vi "Click Cycle.vi"(6 "Prior Property Selection":T1(array[cluster]), 7 "Action":T2, 8 "Shift":bool, 9 "Coords":cluster{"Horizontal":i32, "Vertical":i32}, 10 "All Tree Refs":refnum<vi>[](array[refnum]), 11 "Tree Control Ref":refnum<vi>) -> (0 "Error Out":errorcluster, 2 "Clicked disabled item?":bool)   [LabVIEW 2023]
doc: "Toggle symbol (R/W) for clicked items in tree."
uses:
  controls/action enum.ctl
panel:
  out "Tag Selected":string[](array[string])
  in  "error in":errorcluster
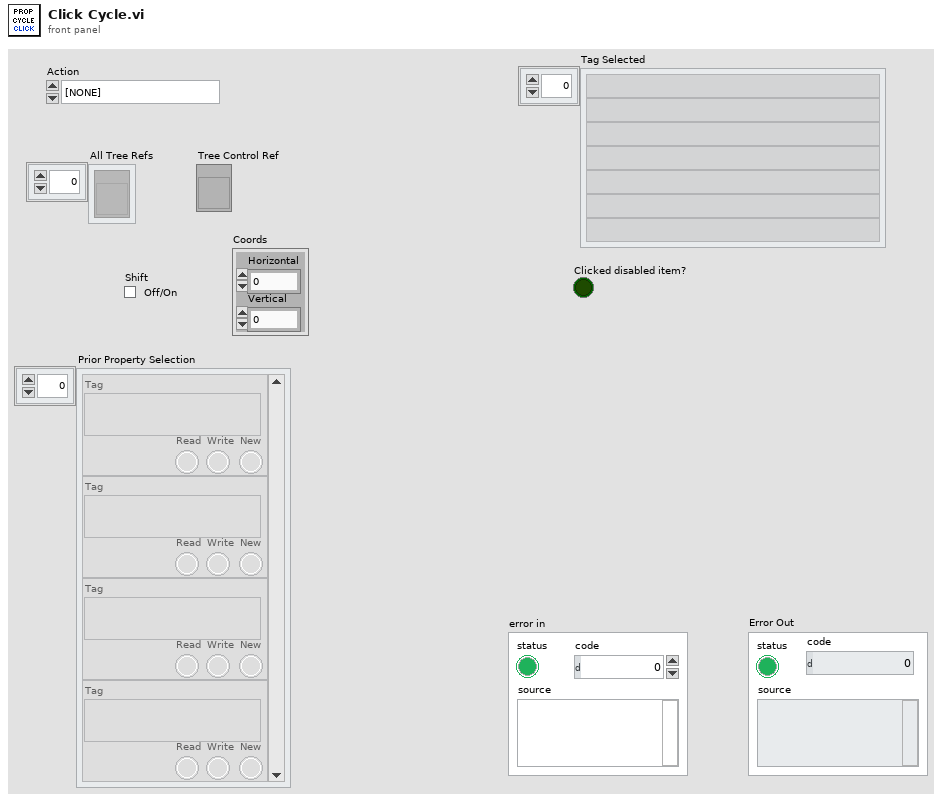
[diagram p1: front panel]
types:
  T1 = cluster{"Tag":string, "Read":bool, "Write":bool, "New":bool}[]
  T2 = typedef "action enum.ctl" = enum16{"[NONE]", "APP_SEPARATOR", "Wire Bundle", "Wire Unbundle", "Terminal Unbundle", "Terminal Bundle", "Bundler Move Up", "Bundler Move Down", "Bundler Insert", "Bundler Remove", "Bundler Remove Unwired", "Bundler Rearrange", "In Place Insert", "In Place Remove", "In Place Remove Unwired", "In Place Rearrange", "Wire Properties", "Wire Method", "Terminal Properties", "Terminal Method", "Property Move Up", "Property Move Down", "Properties Insert", "Properties Remove", "Properties Remove Unwired", "Properties Rearrange", "Method Change", "Class For Constant", "Class For Control", "Class For Node", "Class Name to Clipboard"}
  T3 = cluster{"Can R":bool, "Can W":bool, "Is R":bool, "Is W":bool}
  T4 = enum16{"Init", "Read", "Remove", "Remove or Append", "Append", "Append If New"}
  T5 = cluster{"Index":u16, "Property Type":enum16{"Unknown", "Base", "Scripting", "Private", "Deprecated", "None", "Divider"}, "ID String":string, "Dotted ID String":string, "Class":string, "Parent":string, "Display name full":string, "Display name short":string, "Parents Array":string[], "Indent":u16}
  T6 = enum16{"Unknown", "Base", "Scripting", "Private", "Deprecated", "None", "Divider"}
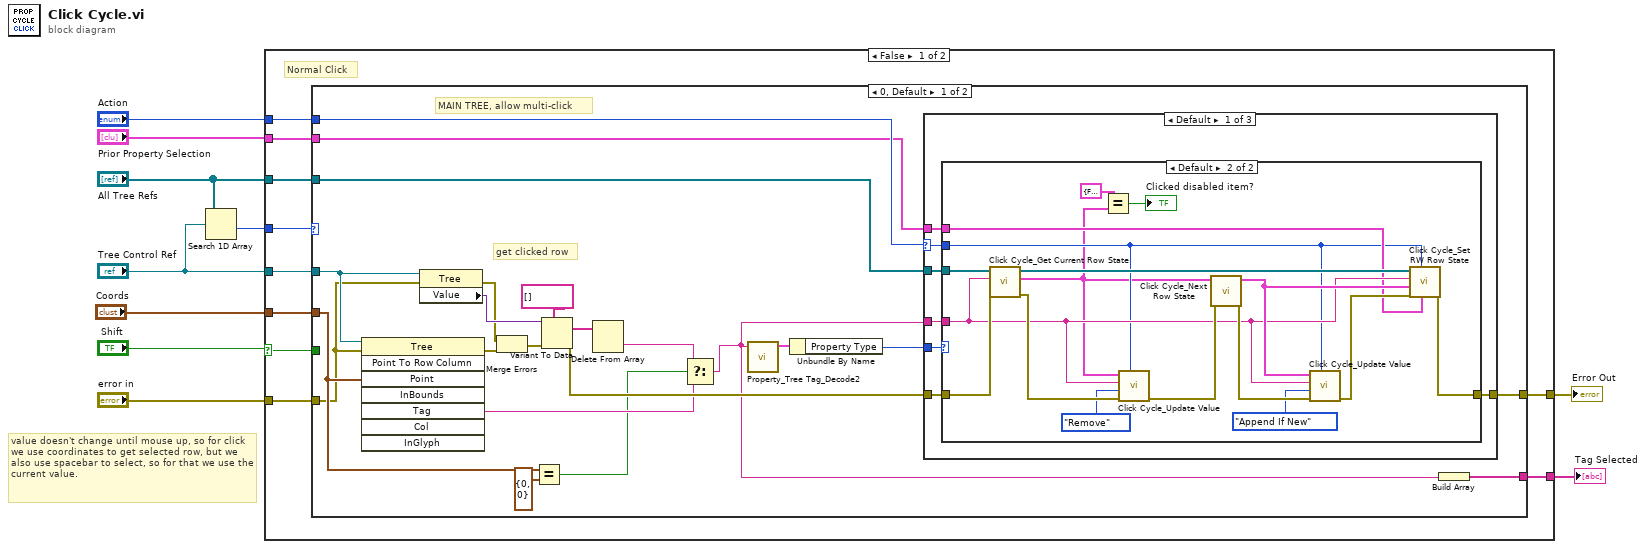
[diagram p0: block diagram]
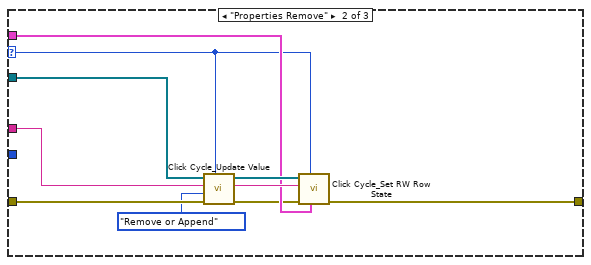
[diagram p3: hidden frame]
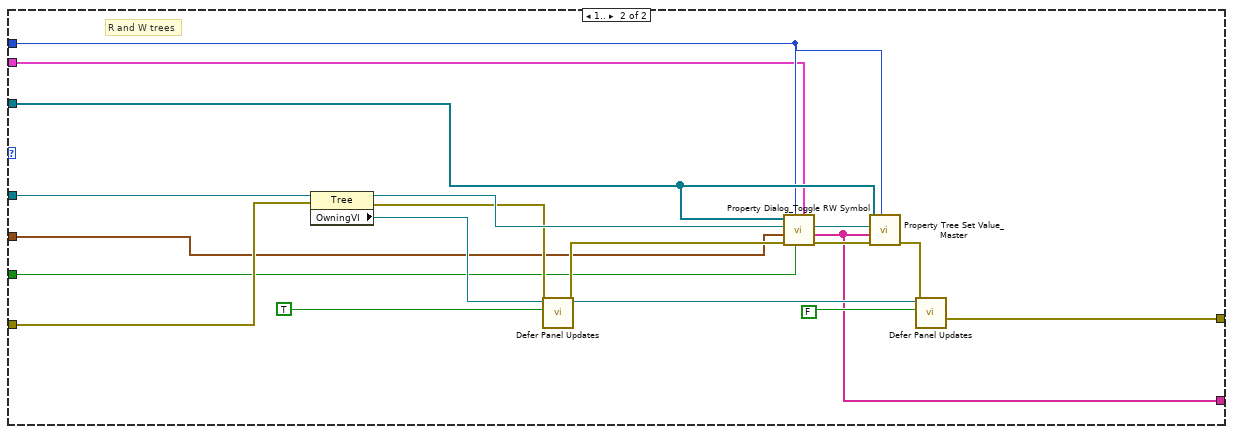
[diagram p5: hidden frame]
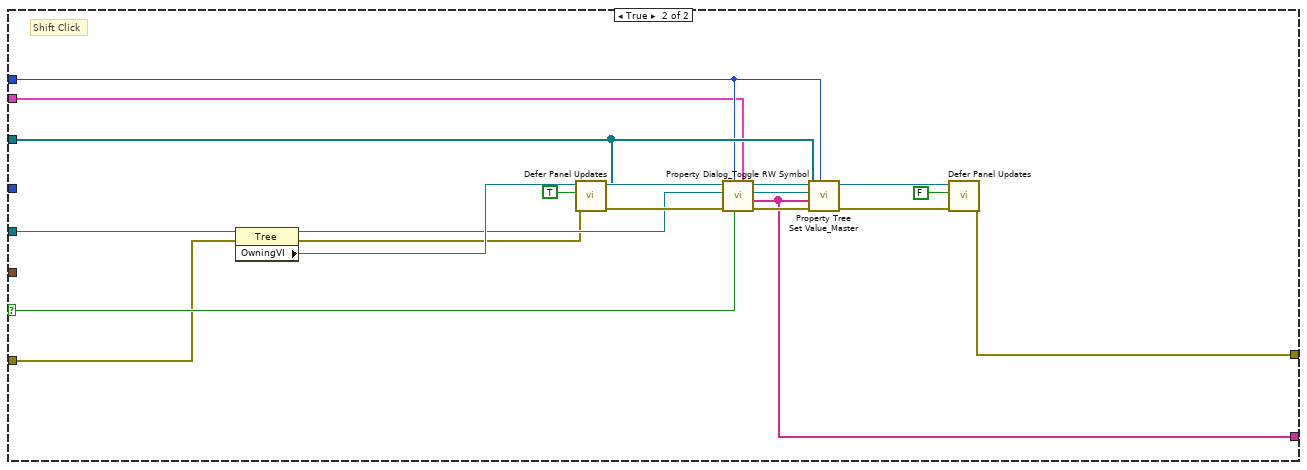
[diagram p6: hidden frame]
diagram:
  # "value doesn't change until mouse up, so for click we use coordinates to get selected row, but we also use spacebar to select, so for that we use the current value."
  n1 = Search 1D Array(1D array="All Tree Refs", element="Tree Control Ref") -> (index of element=w4:i32)  [unwired: 1 in]
  n2 = case shown="False" "Shift" {
    selector: "Shift" -> [w13 w99]
    tunnel: "error in" -> [w20 w96]
    tunnel: "All Tree Refs" -> [w19 w101]
    tunnel: "Tree Control Ref" -> [w18 w106]
    tunnel: w4 -> [w15 _]
    tunnel: [w17 w104] -> w7
    tunnel: [w16 w103] -> w6
    tunnel: "Action" -> [w14 w100]
    tunnel: "Prior Property Selection" -> [w12 w98]
    tunnel: "Coords" -> [w11 _]
    frame False {
      # "Normal Click"
      n3 = case shown="0, Default" w15 {
        tunnel: w20 -> [w21 w84]
        tunnel: w19 -> [w42 w86]
        tunnel: w18 -> [w31 w85]
        tunnel: [w41 w82] -> w17
        tunnel: [w40 w81] -> w16
        tunnel: w14 -> [w37 w79]
        tunnel: w13 -> [_ w80]
        tunnel: w12 -> [w36 w78]
        tunnel: w11 -> [w24 w77]
        frame 0, Default {
          # "MAIN TREE, allow multi-click"
          # "get clicked row"
          n4 = invoke class="Tree" method="Point To Row Column"(reference=w31, error in=w21, "Point"=w24) -> (error out=w28:errorcluster, "Tag"=w25:string)  [unwired: 5 in, 6 out]
          n5 = property class="Tree"(reference=w31, error in=w21) -> (error out=w27:errorcluster, "Value"=w35:variant)  [unwired: 1 out]
          n6 = Merge Errors(w27, w28) -> (w26:errorcluster)
          n7 = Equal?(x=w24, y=cluster{"Horizontal":i32, "Vertical":i32} {"Horizontal"=0, "Vertical"=0} ("Coords")) -> (x = y?=w22:bool)
          n8 = Variant To Data(error in=w26, type=string[] [], Variant=w35) -> (data=w33:string[], error out=w32:errorcluster)
          n9 = Delete From Array(array=w33) -> (deleted portion=w30:string)  [unwired: 2 in, 1 out]
          n10 = Select(t=w30, s=w22, f=w25) -> (s? t:f=w29:string)
          n11 = call "Property_Tree Tag_Decode2.vi"("Tag In"=w29) -> ("TagData"=w39:T5)  [unwired: 10 in]
          n12 = Unbundle By Name(w39) -> ("Property Type"=w38:T6)
          n13 = case shown="Default" w37 {
            selector: w37 -> [w44 w68 _]
            tunnel: w42 -> [w49 w75 _]
            tunnel: [w48 w74 w76] -> w41
            tunnel: w32 -> [w47 w73 w76]
            tunnel: w29 -> [w46 w72 _]
            tunnel: w38 -> [w45 _ _]
            tunnel: w36 -> [w43 w71 _]
            frame Default {
              n14 = case shown="Default" w45 {
                tunnel: w49 -> [_ w67]
                tunnel: [w50 w66] -> w48
                tunnel: w47 -> [w50 w60]
                tunnel: w46 -> [_ w58]
                tunnel: w44 -> [_ w54]
                tunnel: w43 -> [_ w57]
                frame "Divider" {
                  # "Ignore clicks on Divider"
                }
                frame Default {
                  n15 = call "Click Cycle_Get Current Row State.vi"("error in"=w60, "Active Item:Tag"=w58, "All Tree Refs"=w67) -> ("error out"=w64:errorcluster, "Row RW State"=w53:T3, "All Tree Refs Out"=w61:refnum<vi>[])  [unwired: 6 in]
                  n16 = Equal?(x=T3 {"Can R"=FALSE, "Can W"=FALSE, "Is R"=FALSE, "Is W"=FALSE} ("Row RW State"), y=w53) -> (x = y?=→"Clicked disabled item?":bool)
                  n17 = call "Click Cycle_Update Value.vi"("Action"=w54, "Error In"=w64, "Save Action"=T4."Remove" ("Action"), "Tag"=w58, "Row RW State"=w53) -> ("Error Out"=w63:errorcluster)  [unwired: 6 in]
                  n18 = call "Click Cycle_Next Row State.vi"("Error In"=w63, "Current Row State"=w53) -> ("Error Out"=w62:errorcluster, "Next Row State"=w65:T3)  [unwired: 8 in]
                  n19 = call "Click Cycle_Update Value.vi"("Action"=w54, "Error In"=w62, "Save Action"=T4."Append If New" ("Action"), "Tag"=w58, "Row RW State"=w65) -> ("Error Out"=w59:errorcluster)  [unwired: 6 in]
                  n20 = call "Click Cycle_Set RW Row State.vi"("Prior Property Array"=w57, "Action"=w54, "Error In"=w59, "Row RW State"=w65, "Active Item:Tag"=w58, "All Tree Refs"=w61) -> ("Error Out"=w66:errorcluster)  [unwired: 4 in, 1 out]
                }
              }
            }
            frame "Properties Remove" {
              n21 = call "Click Cycle_Update Value.vi"("Action"=w68, "Error In"=w73, "Save Action"=T4."Remove or Append" ("Action"), "Tag"=w72) -> ("Error Out"=w70:errorcluster)  [unwired: 7 in]
              n22 = call "Click Cycle_Set RW Row State.vi"("Prior Property Array"=w71, "Action"=w68, "Error In"=w70, "Active Item:Tag"=w72, "All Tree Refs"=w75) -> ("Error Out"=w74:errorcluster)  [unwired: 5 in, 1 out]
            }
            frame "Properties Rearrange" {
            }
          }
          n23 = Build Array(w29) -> (w40:string[])
        }
        frame 1.. {
          # "R and W trees"
          n24 = property class="Tree"(reference=w85, error in=w84) -> (reference out=w89:refnum<vi>, error out=w83:errorcluster, "OwningVI"=w90:refnum<vi>)
          n25 = call "Defer Panel Updates.vi"("error in (no error)"=w83, "Defer Panel Updates [T]"=TRUE, "VI Ref"=w90) -> ("error out"=w94:errorcluster, "VI Ref Out"=w93:refnum<vi>)  [unwired: 7 in]
          n26 = call "Property Dialog_Toggle RW Symbol.vi"("Prior Property Array"=w78, "Shift click?"=w80, "Action"=w79, "Error In"=w94, "Coords"=w77, "Tree Control in"=w89, "All Tree Refs"=w86) -> ("Error Out"=w92:errorcluster, "Tag Selected"=w81:string[], "Tree Control Out"=w91:refnum<vi>)  [unwired: 2 in]
          n27 = call "Property Tree Set Value_Master.vi"("Action"=w79, "Error In"=w92, "Tag Selected"=w81, "Active Tree"=w91, "All Tree Refs"=w86) -> ("Error Out"=w95:errorcluster)  [unwired: 6 in]
          n28 = call "Defer Panel Updates.vi"("error in (no error)"=w95, "Defer Panel Updates [T]"=FALSE, "VI Ref"=w93) -> ("error out"=w82:errorcluster)  [unwired: 7 in, 1 out]
        }
      }
    }
    frame True {
      # "Shift Click"
      n29 = property class="Tree"(reference=w106, error in=w96) -> (reference out=w102:refnum<vi>, error out=w97:errorcluster, "OwningVI"=w105:refnum<vi>)
      n30 = call "Defer Panel Updates.vi"("error in (no error)"=w97, "Defer Panel Updates [T]"=TRUE, "VI Ref"=w105) -> ("error out"=w112:errorcluster, "VI Ref Out"=w111:refnum<vi>)  [unwired: 7 in]
      n31 = call "Property Dialog_Toggle RW Symbol.vi"("Prior Property Array"=w98, "Shift click?"=w99, "Action"=w100, "Error In"=w112, "Tree Control in"=w102, "All Tree Refs"=w101) -> ("Error Out"=w108:errorcluster, "Tag Selected"=w103:string[], "Tree Control Out"=w107:refnum<vi>)  [unwired: 3 in]
      n32 = call "Property Tree Set Value_Master.vi"("Action"=w100, "Error In"=w108, "Tag Selected"=w103, "Active Tree"=w107, "All Tree Refs"=w101) -> ("Error Out"=w113:errorcluster)  [unwired: 6 in]
      n33 = call "Defer Panel Updates.vi"("error in (no error)"=w113, "Defer Panel Updates [T]"=FALSE, "VI Ref"=w111) -> ("error out"=w104:errorcluster)  [unwired: 7 in, 1 out]
    }
  }
  "Error Out" <- w7
  "Tag Selected" <- w6
